vi "Init.vi"(8 "error in (no error)":errorcluster, 10 "IConfigure":refnum<class "IConfigure.lvclass">, 11 "IInstrument Base in":refnum<class "IInstrument Base.lvclass">) -> (0 "error out":errorcluster, 3 "IInstrument Base out":refnum<class "IInstrument Base.lvclass">)   [LabVIEW 2023, in "HAL Interfaces.lvlib" / "IInstrument Base.lvclass"]
uses:
  IInstrument Base.lvclass
  IConfigure/IConfigure.lvclass
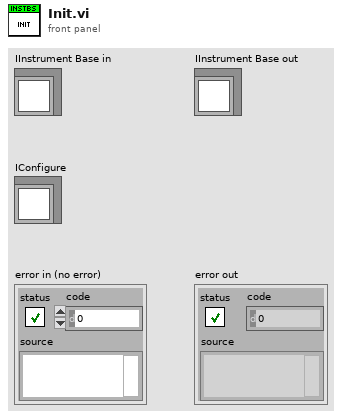
[diagram p1: front panel]
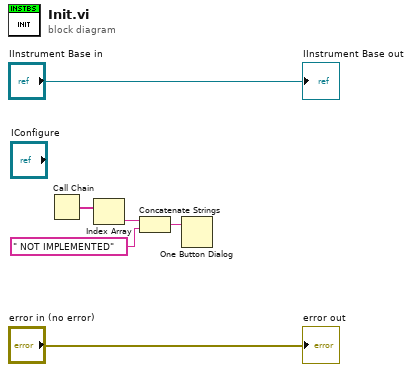
[diagram p0: block diagram]
diagram:
  n1 = Call Chain() -> (call chain=w4:string[])
  n2 = Index Array(array=w4) -> (element=w1:string)  [unwired: 1 in]
  n3 = Concatenate Strings(w1, " NOT IMPLEMENTED" ("string")) -> (w3:string)
  n4 = One Button Dialog(message=w3) -> ()  [unwired: 1 in, 1 out]
  "error out" <- "error in (no error)"
  "IInstrument Base out" <- "IInstrument Base in"
